vi "End Scripting Session.vi"(8 "error in":errorcluster, 10 "Scripting Session":T1, 11 "VI in":refnum<vi>) -> (0 "error out":errorcluster, 3 "VI out":refnum<vi>)   [LabVIEW 2020, in "Enclose in Structure.lvlib"]
uses:
  Enclose in Structure.lvlib
  Scripting Session.ctl
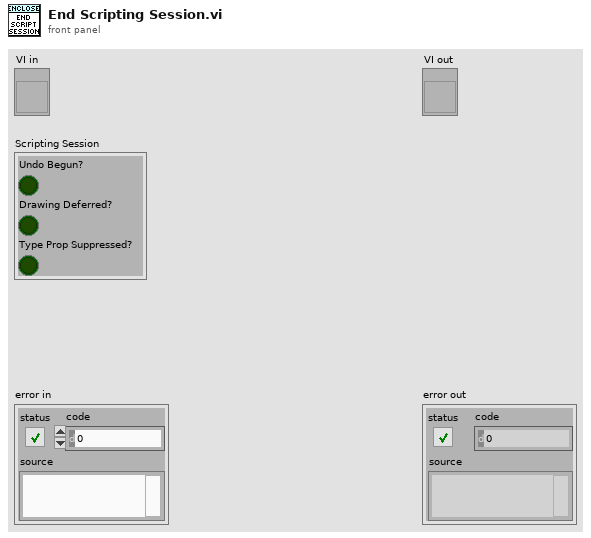
[diagram p1: front panel]
types:
  T1 = typedef "Enclose in Structure.lvlib/Scripting Session.ctl" = cluster{"Undo Begun?":bool, "Drawing Deferred?":bool, "Type Prop Suppressed?":bool}
  T2 = typedef "LVPointTypeDef.ctl" = cluster{"Horizontal":i16, "Vertical":i16}
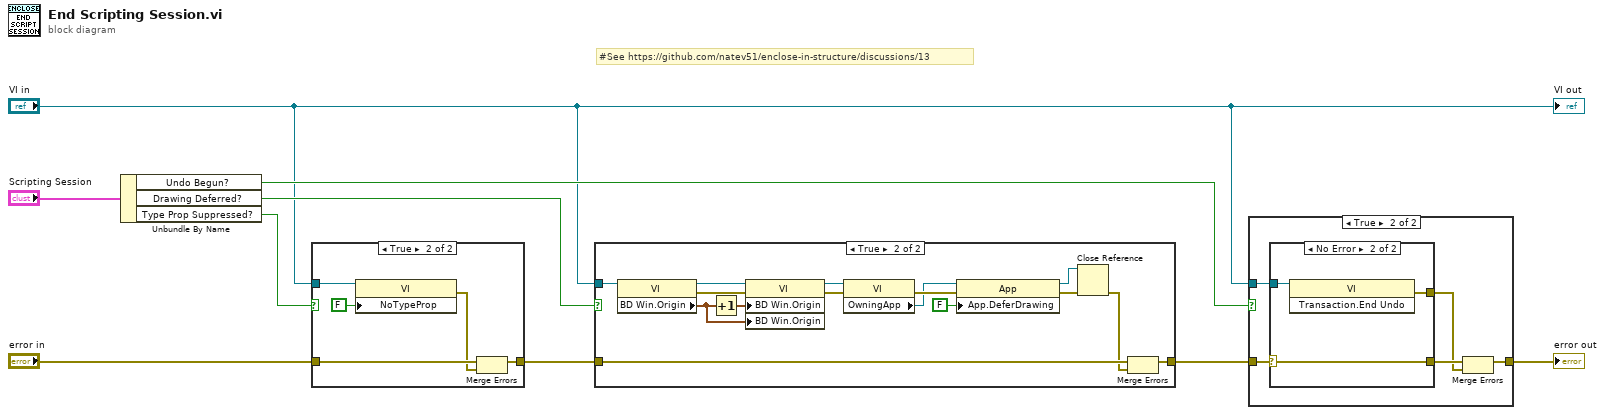
[diagram p0: block diagram]
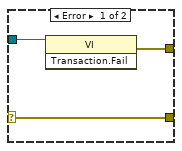
[diagram p3: hidden frame]
diagram:
  # "#See https://github.com/natev51/enclose-in-structure/discussions/13"
  n1 = Unbundle By Name("Scripting Session") -> ("Undo Begun?"=w4:bool, "Drawing Deferred?"=w5:bool, "Type Prop Suppressed?"=w8:bool)
  n2 = case shown="True" w8 {
    tunnel: "VI in" -> [_ w15]
    tunnel: "error in" -> [w10 w13]
    tunnel: [w10 w11] -> w6
    frame False {
    }
    frame True {
      n3 = property class="VI"(reference=w15, "NoTypeProp"=FALSE ("Suppress Type Prop")) -> (error out=w12:errorcluster)  [unwired: 1 in, 1 out]
      n4 = Merge Errors(w13, w12) -> (w11:errorcluster)
    }
  }
  n5 = case shown="True" w5 {
    tunnel: w6 -> [w16 w31]
    tunnel: [w16 w30] -> w3
    tunnel: "VI in" -> [_ w19]
    frame False {
    }
    frame True {
      n6 = property class="VI"(reference=w19) -> (reference out=w22:refnum<vi>, error out=w21:errorcluster, "BD Win.Origin"=w18:T2)  [unwired: 1 in]
      n7 = Increment(x=w18) -> (x+1=w23:T2)
      n8 = property class="VI"(reference=w22, error in=w21, "BD Win.Origin"=w23, "BD Win.Origin"=w18) -> (reference out=w20:refnum<vi>, error out=w17:errorcluster)
      n9 = property class="VI"(reference=w20, error in=w17) -> (error out=w29:errorcluster, "OwningApp"=w28:refnum<vi>)  [unwired: 1 out]
      n10 = property class="App"(reference=w28, error in=w29, "App.DeferDrawing"=FALSE ("Application:Defer Drawing")) -> (reference out=w24:refnum<vi>, error out=w26:errorcluster)
      n11 = Close Reference(reference=w24, error in (no error)=w26) -> (error out=w25:errorcluster)
      n12 = Merge Errors(w31, w25) -> (w30:errorcluster)
    }
  }
  n13 = case shown="True" w4 {
    tunnel: [w32 w34] -> w2
    tunnel: "VI in" -> [_ w36]
    tunnel: w3 -> [w32 w35]
    frame False {
    }
    frame True {
      n14 = case shown="No Error" w35 {
        selector: w35 -> [w39 w41]
        tunnel: w36 -> [w40 w43]
        tunnel: [w38 w42] -> w33
        tunnel: [w39 w41] -> w37
        frame Error {
          n15 = invoke class="VI" method="Transaction.Fail"(reference=w40) -> (error out=w38:errorcluster)  [unwired: 2 in, 2 out]
        }
        frame No Error {
          n16 = invoke class="VI" method="Transaction.End Undo"(reference=w43) -> (error out=w42:errorcluster)  [unwired: 2 in, 2 out]
        }
      }
      n17 = Merge Errors(w37, w33) -> (w34:errorcluster)
    }
  }
  "error out" <- w2
  "VI out" <- "VI in"
